vi "9.1.vi"() -> ()   [LabVIEW 2017]
panel:
  out "sum":dbl
  out "size(s)":i32
  in  "String":string
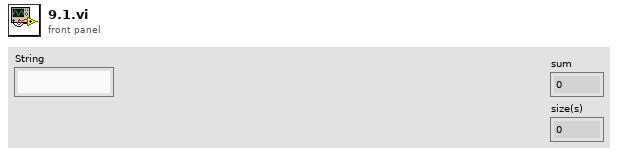
[diagram p1: front panel]
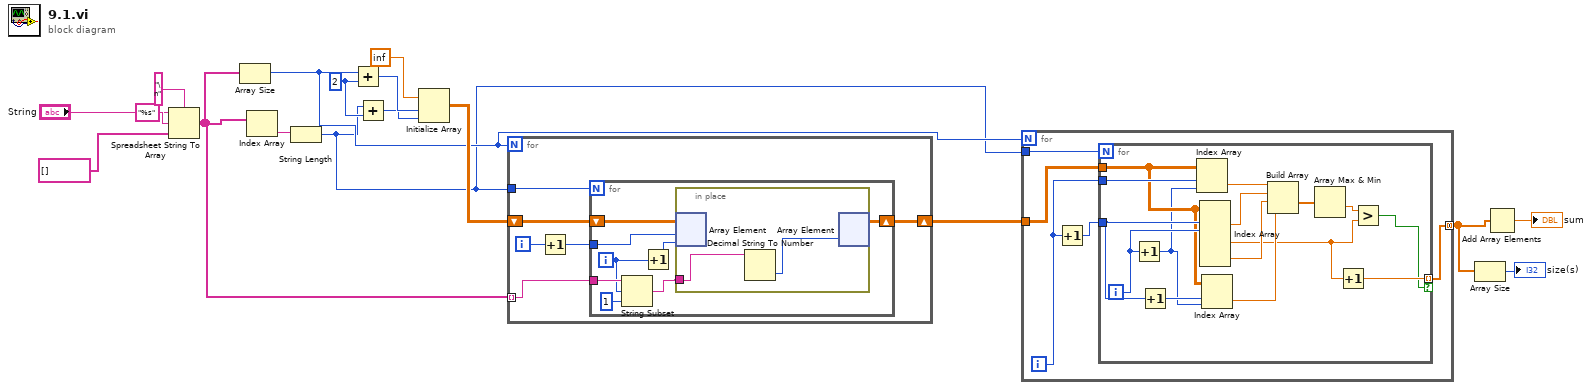
[diagram p0: block diagram]
diagram:
  w12 = 2 ("y")
  n1 = Spreadsheet String To Array(delimiter (Tab)="\n", format string="%s", spreadsheet string="String", array type (2D Dbl)=string[] []) -> (array=w7:string[])
  n2 = Array Size(array=w7) -> (size(s)=w5:i32)
  n3 = Index Array(array=w7) -> (element=w13:string)  [unwired: 1 in]
  n4 = String Length(string=w13) -> (length=w4:i32)
  n5 = Add(x=w5, y=w12) -> (x+y=w11:i32)
  n6 = Add(x=w4, y=w12) -> (x+y=w10:i32)
  n7 = Initialize Array(inf ("element"), w11, w10) -> (w8:dbl[][])
  n8 = for {
    N: w5 -> [_]
    tunnel: w4 -> [w23]
    shift-right: [w21] -> w6
    shift-left: w8 -> [w22]
    tunnel: w7 -> [w18] mode=indexing
    i -> [w19]
    n9 = Increment(x=w19) -> (x+1=w20:i32)
    n10 = for {
      N: w23 -> [_]
      shift-right: [w26] -> w21
      shift-left: w22 -> [w31]
      tunnel: w20 -> [w30]
      tunnel: w18 -> [w28]
      i -> [w24]
      n11 = String Subset(string=w28, offset (0)=w24, length (rest)=1 ("length (rest)")) -> (substring=w27:string)
      n12 = Increment(x=w24) -> (x+1=w25:i32)
      n13 = in-place {
        in-place-border: w27 -> [w33]
        n14 = in-place-array #1(w31, w30, w25) -> ()  [unwired: 1 out]
        n15 = Decimal String To Number(string=w33) -> (number=w32:i32)  [unwired: 2 in, 1 out]
        n16 = in-place-array #1(w32) -> (w26:dbl[][])  [unwired: 2 out]
      }
    }
  }
  n17 = for {
    N: w5 -> [_]
    tunnel: w6 -> [w36]
    tunnel: w4 -> [w38]
    tunnel: [w34] -> w2 mode=concatenating
    i -> [w37]
    n18 = Increment(x=w37) -> (x+1=w35:i32)
    n19 = for {
      N: w38 -> [_]
      tunnel: w37 -> [w53]
      tunnel: w36 -> [w50]
      tunnel: w35 -> [w52]
      tunnel: [w42] -> w34 mode=indexing if=w39
      i -> [w51]
      n20 = Increment(x=w51) -> (x+1=w48:i32)
      n21 = Increment(x=w52) -> (x+1=w49:i32)
      n22 = Index Array(array=w50, index (row)=w53, index (col)=w48) -> (element=w47:dbl)
      n23 = Index Array(array=w50, index (row) #1=w52, index (col) #1=w51) -> (element #1=w46:dbl, element #2=w40:dbl, element #3=w45:dbl)  [unwired: 4 in]
      n24 = Index Array(array=w50, index (row)=w49, index (col)=w48) -> (element=w44:dbl)
      n25 = Build Array(w47, w46, w45, w44) -> (w43:dbl[])
      n26 = Array Max & Min(array=w43) -> (min value=w41:dbl)  [unwired: 3 out]
      n27 = Increment(x=w40) -> (x+1=w42:dbl)
      n28 = Greater?(x=w41, y=w40) -> (0:w39:bool)
    }
  }
  n29 = Array Size(array=w2) -> (size(s)=→"size(s)":i32)
  n30 = Add Array Elements(numeric array=w2) -> (sum=→"sum":dbl)
